vi "FTW-Math-Statistics.vi"(0 "Array of Samples":dbl[](array[numeric])) -> (4 "mean":dbl, 6 "max":dbl, 8 "min":dbl, 10 "standard deviation":dbl, 15 "N":i32)   [LabVIEW 2015]
doc: "Computes the <B>mean</B>, <B>standard deviation</B>, and <B>variance</B> of the values in the input sequence <B>X</B>."
panel:
  # "Inputs"
  # "Outputs"
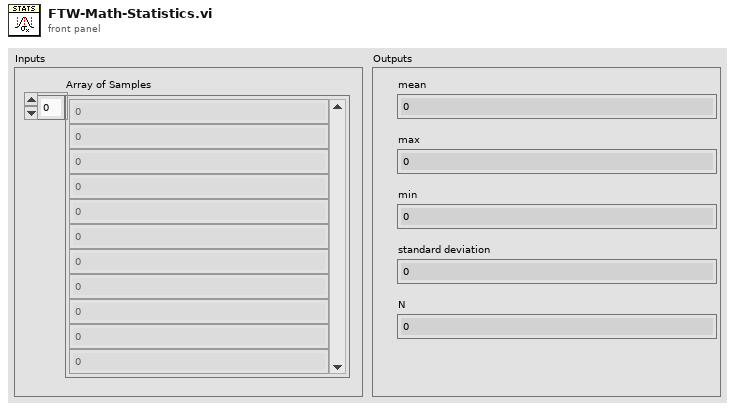
[diagram p1: front panel]
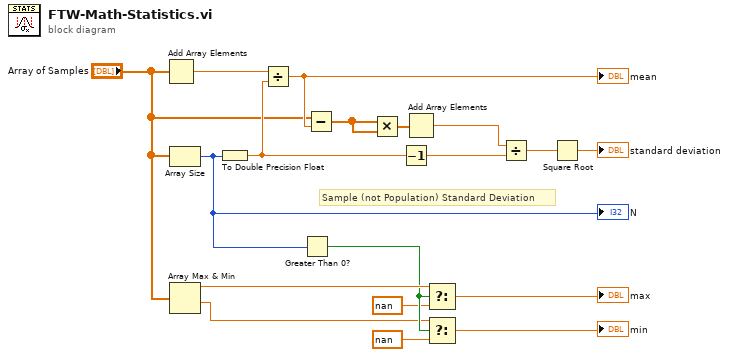
[diagram p0: block diagram]
diagram:
  # "Sample (not Population) Standard Deviation"
  n1 = Add Array Elements(numeric array="Array of Samples") -> (sum=w17:dbl)
  n2 = Array Size(array="Array of Samples") -> (size(s)=w9:i32)
  "N" <- w9
  n3 = Array Max & Min(array="Array of Samples") -> (max value=w8:dbl, min value=w5:dbl)  [unwired: 2 out]
  n4 = To Double Precision Float(number=w9) -> (double precision float=w16:dbl)
  n5 = Divide(x=w17, y=w16) -> (x/y=w15:dbl)
  "mean" <- w15
  n6 = Greater Than 0?(x=w9) -> (x > 0?=w6:bool)
  n7 = Subtract(x="Array of Samples", y=w15) -> (x-y=w11:dbl[])
  n8 = Multiply(x=w11, y=w11) -> (x*y=w10:dbl[])
  n9 = Decrement(x=w16) -> (x-1=w18:dbl)
  n10 = Add Array Elements(numeric array=w10) -> (sum=w12:dbl)
  n11 = Select(t=w8, s=w6, f=nan) -> (s? t:f=→"max":dbl)
  n12 = Select(t=w5, s=w6, f=nan) -> (s? t:f=→"min":dbl)
  n13 = Divide(x=w12, y=w18) -> (x/y=w13:dbl)
  n14 = Square Root(x=w13) -> (sqrt(x)=→"standard deviation":dbl)
